vi "Init_graphe.vi"() -> ()   [LabVIEW 2013]
uses:
  <vilib>/Utility/miscctls.llb/LVRowAndColumnTypeDef.ctl
  <vilib>/Utility/file.llb/Read From Spreadsheet File (string).vi
panel:
  in  "Bouton Aide":bool
  in  "Quit":bool
  out "horodatage_ok":timestamp
  in  "Fichier données brutes":path
  out "Colonne données brutes":string="0"
  out "Ligne données brutes":string="0"
  out "Noms variables":string[](array[string])
  out "Séparateur fichier brute":string
  in  "Valider":bool
  in  "Nouveau format date":bool
  in  "Formats Date - Heure":string(combo)="\"%Y-%m-%d %H:%M:%S\""
  in  "Convertir Date  - heure":bool
  out "Nb lignes":i32
  in  "Séparateur":u16(ring)=1 items=["", ",", ";", ".", "Tab", "Espace"]
  out "Horodatage_1":timestamp[](array[timestamp]) format="%<%X\n%x>T"
  in  "Horodatage 2":timestamp
  out "Table":string[][](table)
  out "Donnees":dbl[][](array[numeric])
  in  "Bouton vide 2":bool
  # "Facultatif : \nSélectionner la dernière cellule des noms de variables  en appuyant sur la touche CTRL"
  # "Sélectionner la 1ère cellule\ndes noms de variables"
  # "Sélectionner la 1ère cellule\nd'horodatage"
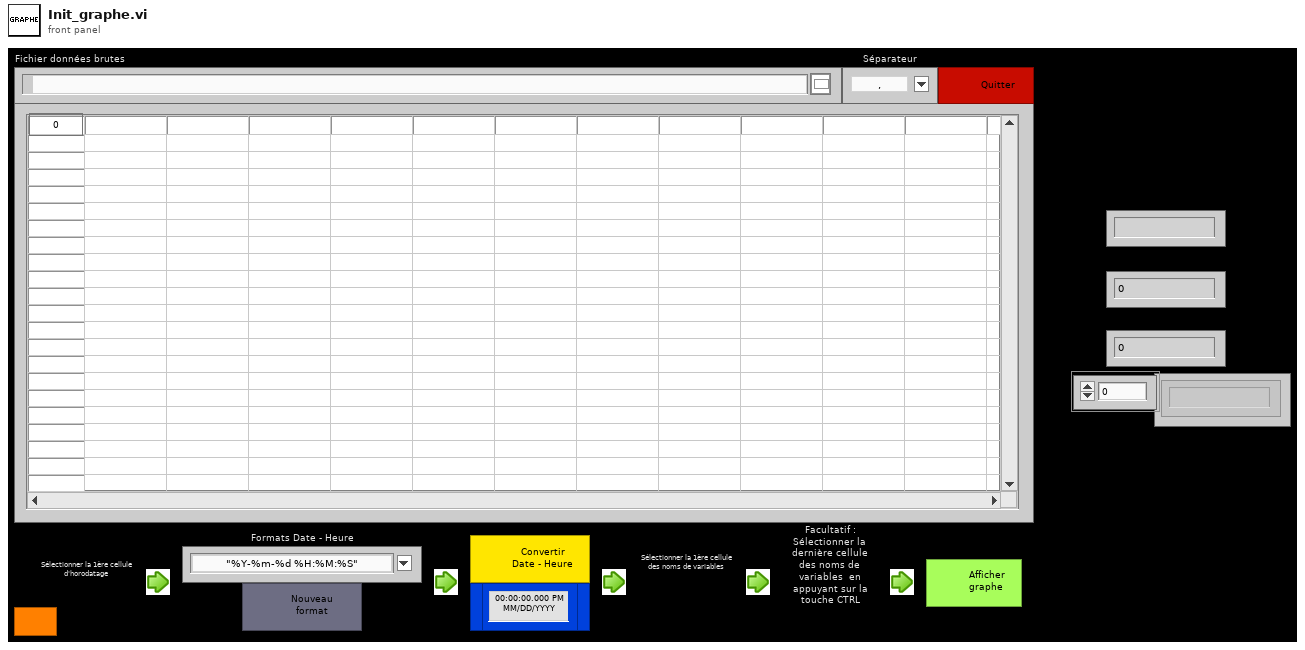
[diagram p1: front panel]
types:
  T1 = typedef "LVRowAndColumnTypeDef.ctl" = cluster{"Row":i32, "Column":i32}
  T2 = typedef "excel Object Reference.ctl" = refnum<k1>
  T3 = enum16{"Left Button", "Center Button", "Right Button", "Window Close"}
  T4 = cluster{"Shift":bool, "Ctrl":bool, "Alt":bool, "Cmd":bool, "Opt":bool}
  T5 = cluster{"Horodatage":timestamp[], "Donnees":dbl[]}[]
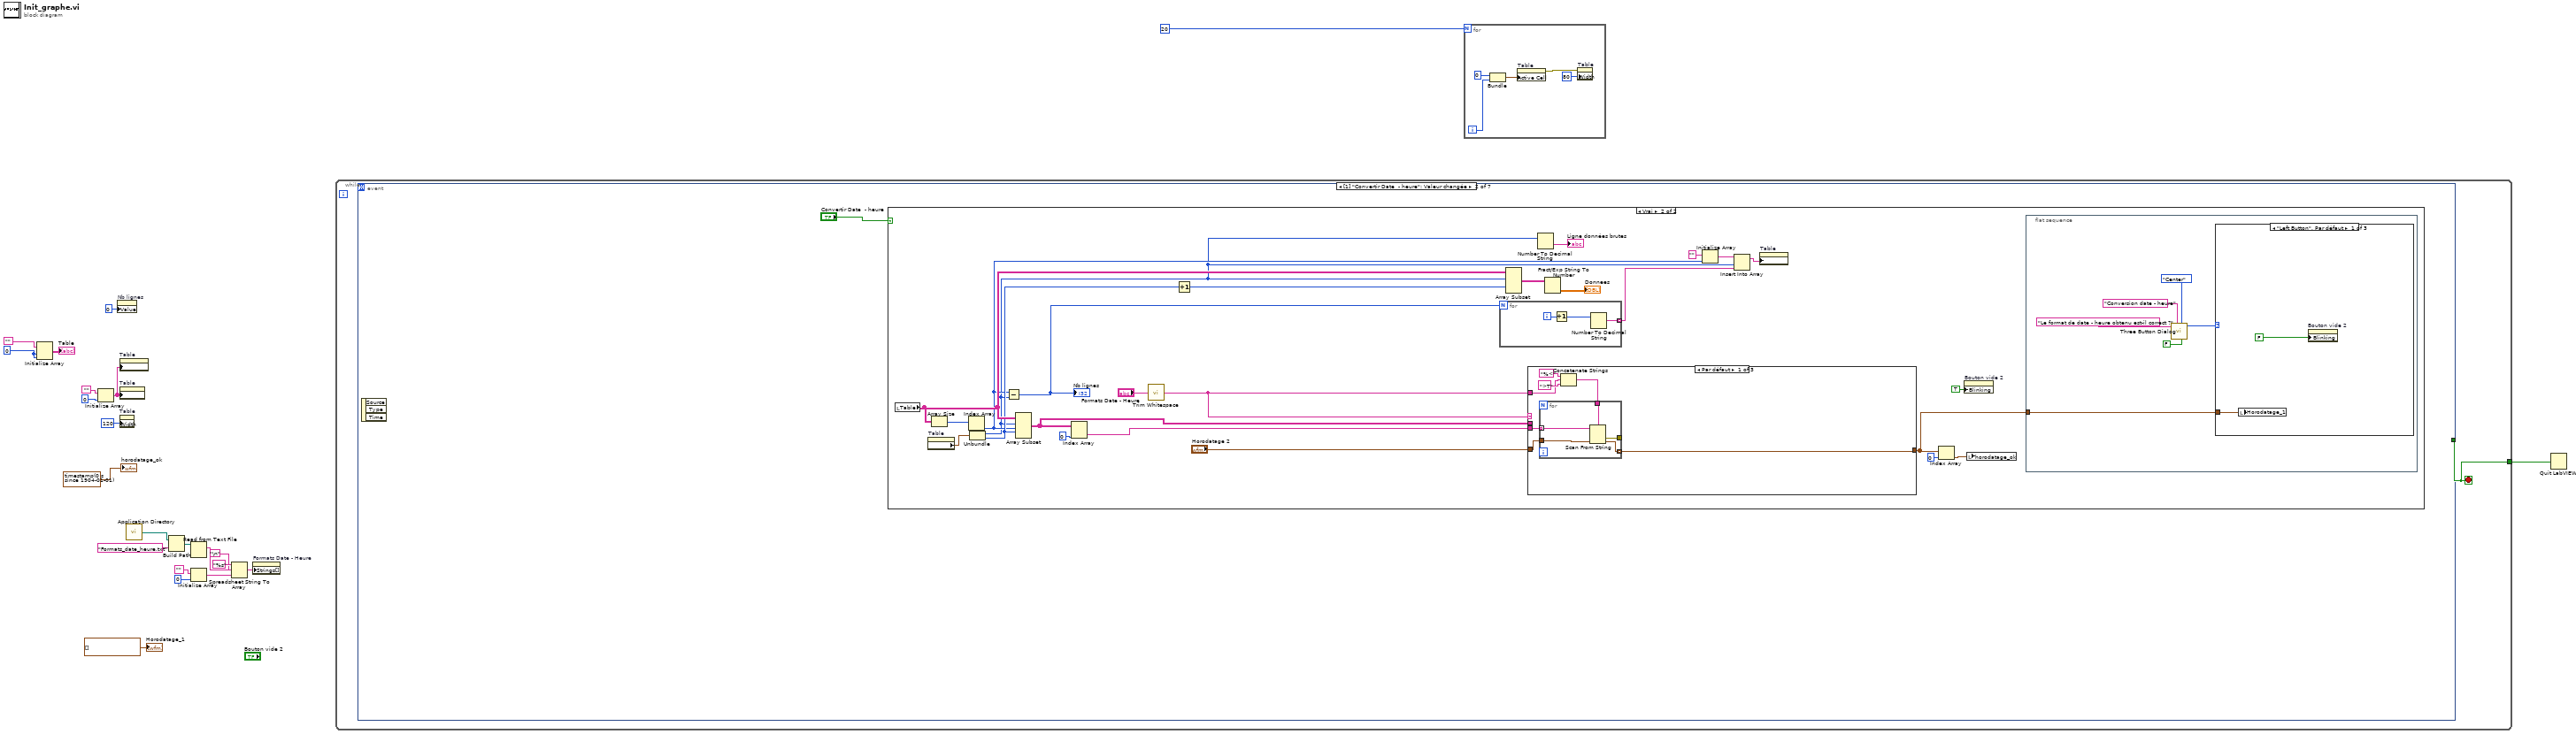
[diagram p0: block diagram]
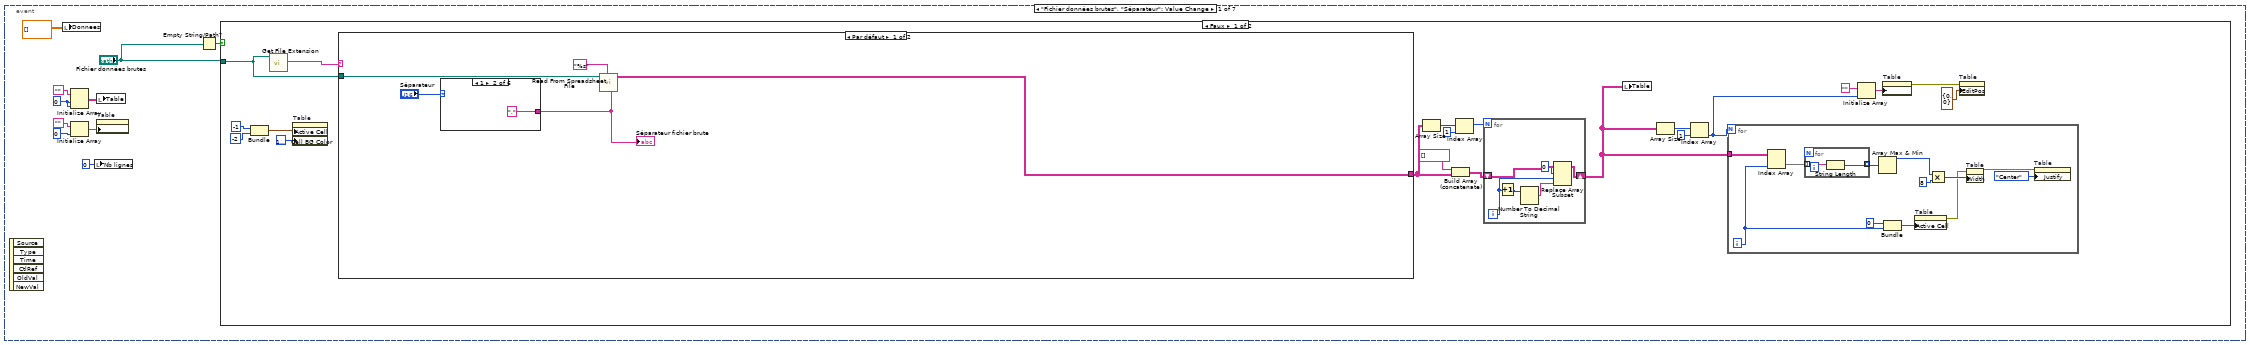
[diagram p2: hidden frame]
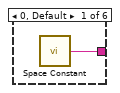
[diagram p3: hidden frame]
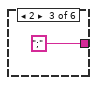
[diagram p4: hidden frame]
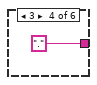
[diagram p5: hidden frame]
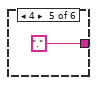
[diagram p6: hidden frame]
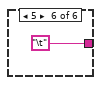
[diagram p7: hidden frame]
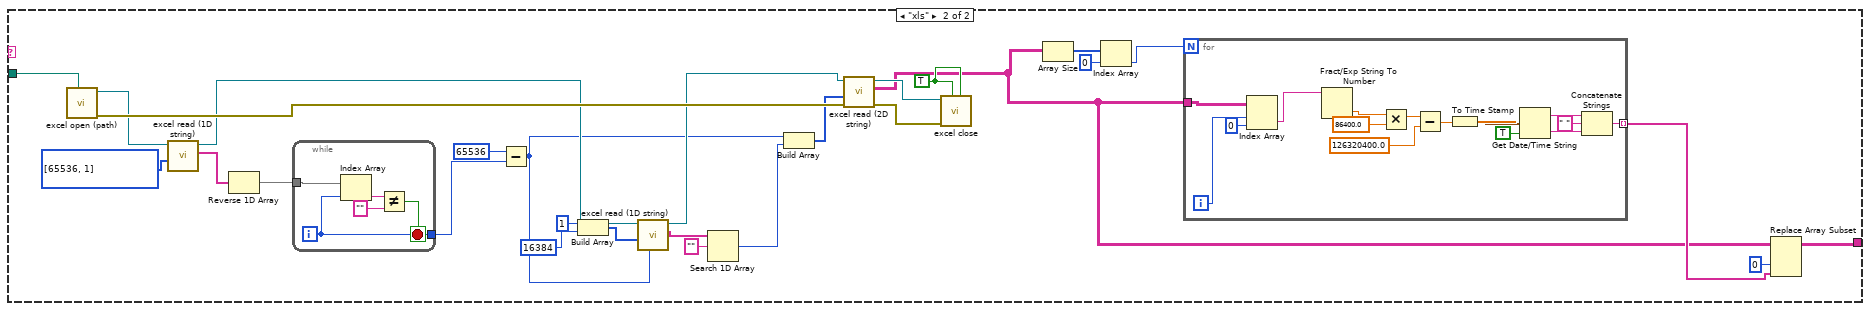
[diagram p8: hidden frame]
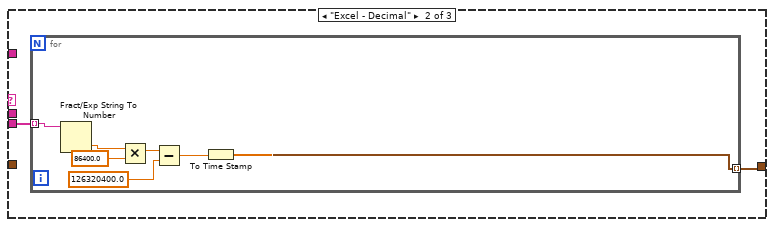
[diagram p13: hidden frame]
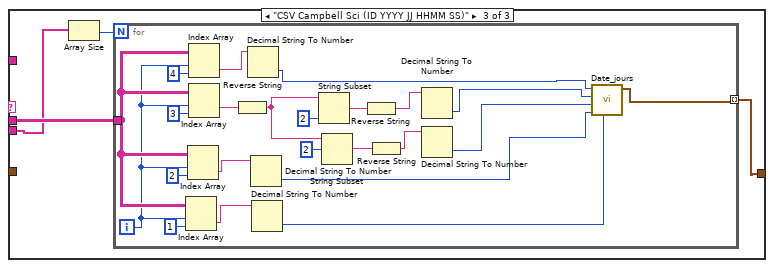
[diagram p14: hidden frame]
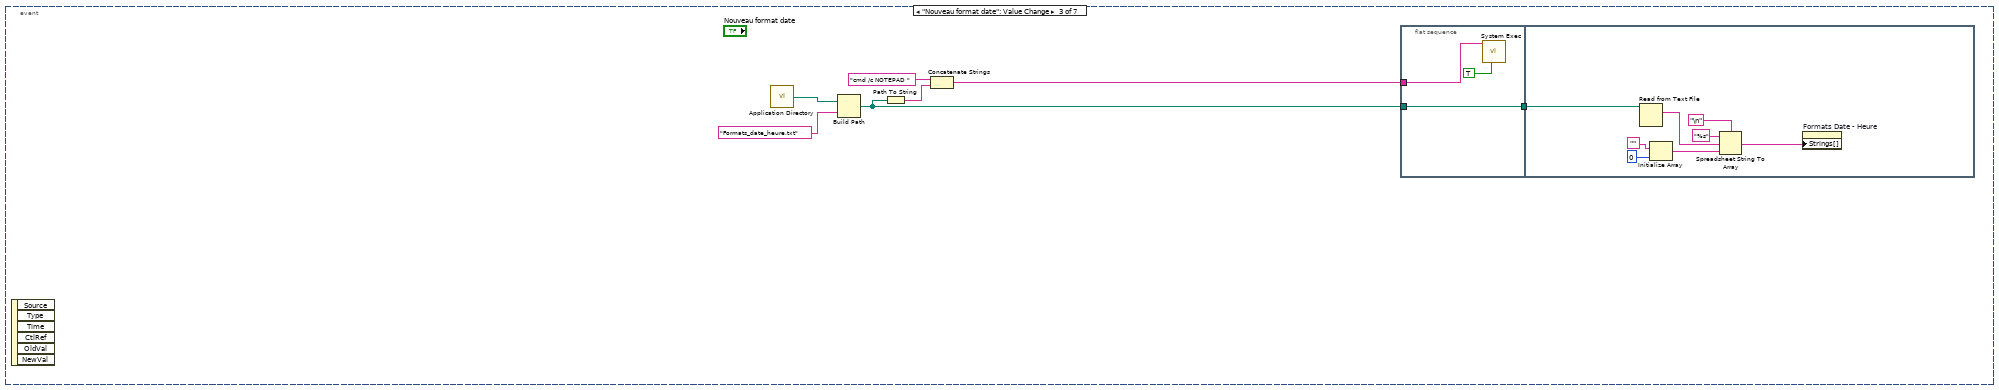
[diagram p15: hidden frame]
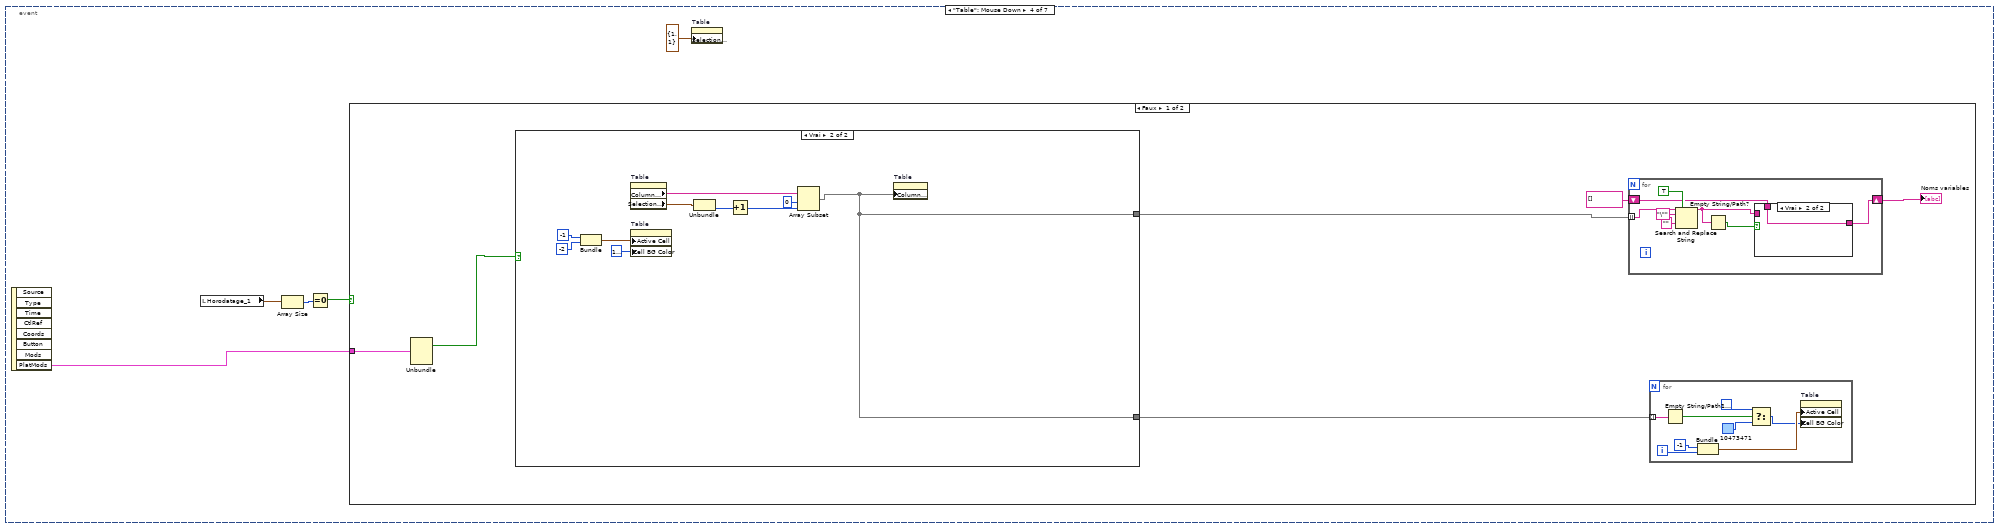
[diagram p16: hidden frame]
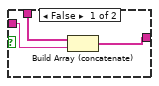
[diagram p17: hidden frame]
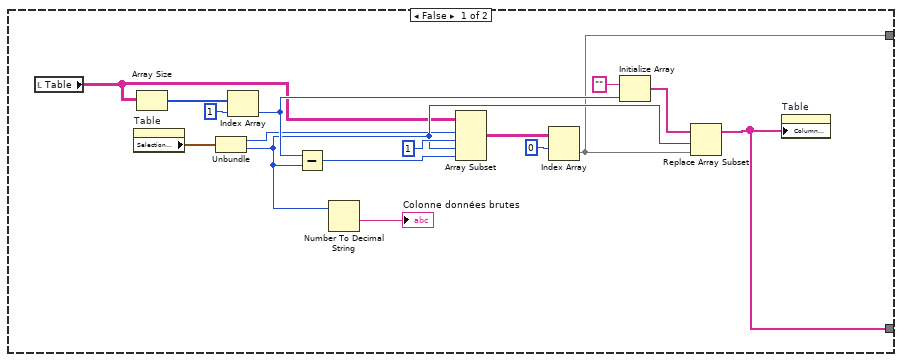
[diagram p18: hidden frame]
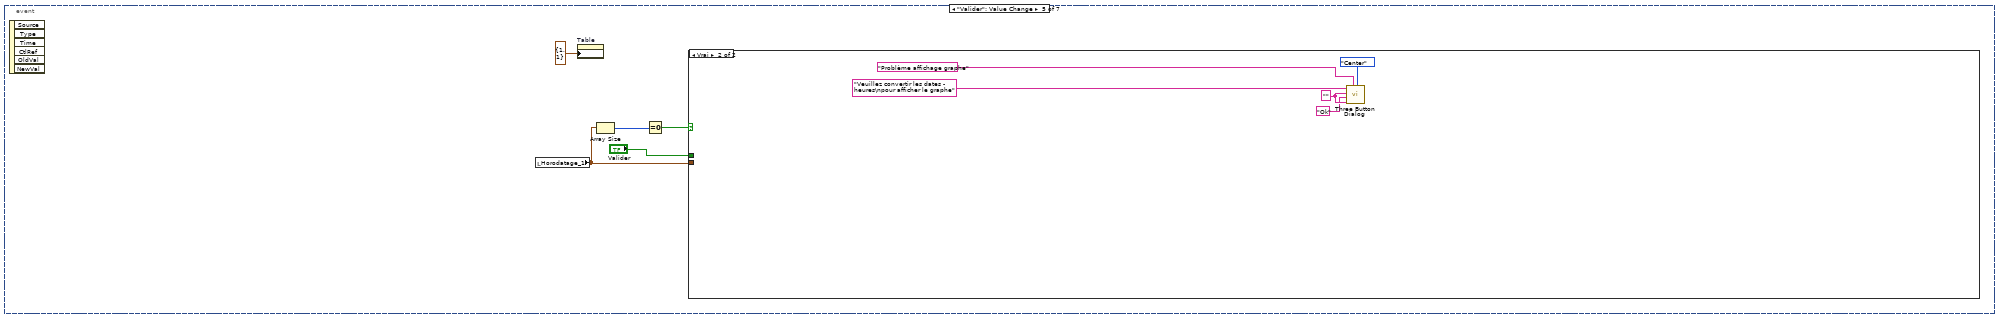
[diagram p20: hidden frame]
diagram:
  w4 = 0 ("taille de la dimension")
  n1 = Initialize Array("", w4, w4) -> (→"Table":string[][])
  n2 = Initialize Array("", 0 ("taille de la dimension")) -> (w11:string[])
  n3 = property on="Nb lignes" class="NumNb (strict)"("Value"=0 ("Nb lignes")) -> ()  [unwired: 2 in, 2 out]
  n4 = property on="Table" class="Tbl (strict)"("Row Headers[]"=w11) -> ()  [unwired: 2 in, 2 out]
  n5 = property on="Table" class="Tbl (strict)"("Column Headers[]"=w11) -> ()  [unwired: 2 in, 2 out]
  n6 = property on="Table" class="Tbl (strict)"("Width"=u32 120 ("Cellule active:Taille de la cellule:Largeur")) -> ()  [unwired: 2 in, 2 out]
  n7 = call <vilib>:"Application Directory.vi"() -> ("Application Directory"=w7:path)
  n8 = Build Path(base path=w7, name or relative path="Formats_date_heure.txt" ("nom ou chemin relatif")) -> (appended path=w15:path)
  n9 = Read from Text File(file (use dialog)=w15) -> (text=w20:string)  [unwired: 3 in, 3 out]
  n10 = Initialize Array("", 0 ("taille de la dimension")) -> (w16:string[])
  n11 = Spreadsheet String To Array(delimiter (Tab)="\n", format string="%s" ("chaîne de format"), spreadsheet string=w20, array type (2D Dbl)=w16) -> (array=w12:string[])
  n12 = property on="Formats Date - Heure" class="ChneDér"("Strings[]"=w12) -> ()  [unwired: 2 in, 2 out]
  n13 = while {
    tunnel: [w23] -> w1
    stop <- w23 stop-if-true
    n14 = event shown="[1] \"Convertir Date  - heure\": Valeur changée" {
      selector: _ -> [_ _ _ _ _ _ _]
      dyn-events: _ -> [_ _ _ _ _ _ _]
      timeout: _ -> [_ _ _ _ _ _ _]
      tunnel: [_ _ _ _ _ w324 _] -> w23
      event "Fichier données brutes", "Séparateur": Value Change {
        w33 = 0 ("taille de la dimension")
        n15 = event-data() -> ()  [unwired: 1 in, 6 out]
        n16 = local write "Donnees"(dbl[][] [] ("Donnees")) -> ()
        n17 = Initialize Array("", w33, w33) -> (w31:string[][])
        n18 = Initialize Array("", 0 ("taille de la dimension")) -> (w28:string[])
        n19 = local write "Nb lignes"(0 ("Nb lignes")) -> ()
        n20 = local write "Table"(w31) -> ()
        n21 = property on="Table" class="Tbl (strict)"("Row Headers[]"=w28) -> ()  [unwired: 2 in, 2 out]
        n22 = Empty String/Path?(string/path="Fichier données brutes") -> (empty?=w25:bool)
        n23 = case shown="Faux" w25 {
          tunnel: "Fichier données brutes" -> [w49 _]
          frame False {
            n24 = Bundle(-1, -2) -> (w44:cluster{i32, i32})  [unwired: 1 in]
            n25 = call <vilib>:"Get File Extension.vi"("file"=w49) -> ("lowercase file extension"=w48:string)  [unwired: 7 in, 3 out]
            n26 = property on="Table" class="Tbl (strict)"("Active Cell"=w44, "Cell BG Color"=u32 16777225) -> ()  [unwired: 2 in, 2 out]
            n27 = case shown="Par défaut" w48 {
              tunnel: w49 -> [w76 w112]
              tunnel: [w75 w85] -> w37
              frame Default {
                n28 = case shown="1" "Séparateur" {
                  tunnel: [w79 "," ";" "." "." "\t"] -> w74
                  frame 0, Default {
                    n29 = call <vilib>:"Space Constant.vi"() -> ("String"=w79:string)
                  }
                  frame 1 {
                  }
                  frame 2 {
                  }
                  frame 3 {
                  }
                  frame 4 {
                  }
                  frame 5 {
                  }
                }
                "Séparateur fichier brute" <- w74
                n30 = call-poly <vilib>:"Read From Spreadsheet File.vi"("delimiter (\\t)"=w74, "format (%s)"="%s", "file path (dialog if empty)"=w76) -> ("all rows"=w75:string[][])  [unwired: 4 in, 4 out]
              }
              frame "xls" {
                w108 = TRUE ("Override closing behavior")
                n31 = call <userlib>:"excel open (path).vi"("workbook path"=w112) -> ("error out"=w109:errorcluster, "reference"=w107:T2)  [unwired: 9 in]
                n32 = call <userlib>:"excel read (1D string).vi"("array size\n  - #rows\n  - #columns"=i32[] [65536, 1] ("array size\n  - #rows\n  - #columns"), "reference"=w107) -> ("1D String Array"=w105:string[], "duplicate reference"=w98:T2)  [unwired: 7 in, 1 out]
                n33 = Reverse 1D Array(array=w105) -> (reversed array=w103:string[])
                n34 = while {
                  tunnel: w103 -> [w132]
                  tunnel: [w128] -> w102
                  i -> [w128]
                  stop <- w129 stop-if-true
                  n35 = Index Array(array=w132, index=w128) -> (element=w131:string)
                  n36 = Not Equal?(x=w131, y="") -> (x != y?=w129:bool)
                }
                n37 = Subtract(x=65536, y=w102) -> (x-y=w95:i32)
                n38 = Build Array(1 ("élément"), 16384 ("élément")) -> (w99:i32[])
                n39 = call <userlib>:"excel read (1D string).vi"("Row"=w95, "array size\n  - #rows\n  - #columns"=w99, "reference"=w98) -> ("1D String Array"=w94:string[], "duplicate reference"=w97:T2)  [unwired: 6 in, 1 out]
                n40 = Search 1D Array(1D array=w94, element="" ("élément")) -> (index of element=w92:i32)  [unwired: 1 in]
                n41 = Build Array(w95, w92) -> (w104:i32[])
                n42 = call <userlib>:"excel read (2D string).vi"("error in (no error)"=w109, "array size\n  - #rows\n  - #columns"=w104, "reference"=w97) -> ("error out"=w110:errorcluster, "2D String Array"=w86:string[][], "duplicate reference"=w111:T2)  [unwired: 6 in]
                n43 = call <userlib>:"excel close.vi"("Close"=w108, "Override closing behavior"=w108, "error in (no error)"=w110, "reference"=w111) -> ()  [unwired: 7 in, 1 out]
                n44 = Array Size(array=w86) -> (size(s)=w88:i32[])
                n45 = Index Array(array=w88, index=0 ("indice")) -> (element=w89:i32)
                n46 = for {
                  N: w89 -> [_]
                  tunnel: w86 -> [w127]
                  tunnel: [w113] -> w91 mode=indexing
                  i -> [w126]
                  n47 = Index Array(array=w127, index (row)=w126, index (col)=0 ("indice désactivé (col)")) -> (element=w114:string)
                  n48 = Fract/Exp String To Number(string=w114) -> (number=w124:dbl)  [unwired: 3 in, 1 out]
                  n49 = Multiply(x=w124, y=86400.0) -> (x*y=w122:dbl)
                  n50 = Subtract(x=w122, y=126320400.0) -> (x-y=w120:dbl)
                  n51 = To Time Stamp(1:w120) -> (0:w119:timestamp)
                  n52 = Get Date/Time String(seconds (now)=w119, want seconds? (F)=TRUE ("secondes ? (F)")) -> (date string=w117:string, time string=w115:string)  [unwired: 1 in]
                  n53 = Concatenate Strings(w117, " " ("chaîne"), w115) -> (w113:string)
                }
                n54 = Replace Array Subset(array=w86, new element=w91, index (col)=0 ("indice désactivé (col)")) -> (w85:string[][])  [unwired: 1 in]
              }
            }
            n55 = Array Size(array=w37) -> (size(s)=w39:i32[])
            n56 = Build Array (concatenate)(string[] [] ("élément"), w37) -> (w35:string[][])
            n57 = Index Array(array=w39, index=1 ("indice")) -> (element=w38:i32)
            n58 = for {
              N: w38 -> [_]
              shift-right: [w59] -> w41
              shift-left: w35 -> [w58]
              i -> [w55]
              n59 = Increment(x=w55) -> (x+1=w57:i32)
              n60 = Number To Decimal String(number=w57) -> (decimal integer string=w54:string)  [unwired: 1 in]
              n61 = Replace Array Subset(array=w58, new element=w54, index (row)=0 ("indice désactivé (ligne)"), index (col)=w55) -> (w59:string[][])
            }
            n62 = local write "Table"(w41) -> ()
            n63 = Array Size(array=w41) -> (size(s)=w47:i32[])
            n64 = Index Array(array=w47, index=1 ("indice")) -> (element=w34:i32)
            n65 = for {
              N: w34 -> [_]
              tunnel: w41 -> [w71]
              i -> [w63]
              n66 = Index Array(array=w71, index (col)=w63) -> (element=w68:string[])  [unwired: 1 in]
              n67 = for {
                tunnel: w68 -> [w73] mode=indexing
                tunnel: [w72] -> w67 mode=indexing
                n68 = String Length(string=w73) -> (length=w72:i32)
              }
              n69 = Array Max & Min(array=w67) -> (max value=w66:i32)  [unwired: 3 out]
              n70 = Bundle(0, w63) -> (w65:cluster{i32, i32})  [unwired: 1 in]
              n71 = property on="Table" class="Tbl (strict)"("Active Cell"=w65) -> (error out=w64:errorcluster)  [unwired: 2 in, 1 out]
              n72 = Multiply(x=w66, y=8) -> (x*y=w70:i32)
              n73 = property on="Table" class="Tbl (strict)"(error in=w64, "Width"=w70) -> (error out=w61:errorcluster)  [unwired: 1 in, 1 out]
              n74 = property on="Table" class="Tbl (strict)"(error in=w61, "Justify"=enum16{"Left", "Center", "Right"}."Center" ("Cellule active:Justification de la cellule")) -> ()  [unwired: 1 in, 2 out]
            }
            n75 = Initialize Array("", w34) -> (w52:string[])
            n76 = property on="Table" class="Tbl (strict)"("Column Headers[]"=w52) -> (error out=w50:errorcluster)  [unwired: 2 in, 1 out]
            n77 = property on="Table" class="Tbl (strict)"(error in=w50, "EditPos"=T1 {"Row"=0, "Column"=0} ("Cellule active:Cellule active")) -> ()  [unwired: 1 in, 2 out]
          }
          frame True {
          }
        }
      }
      event "Convertir Date  - heure": Value Change {
        n78 = event-data() -> ()  [unwired: 1 in, 3 out]
        n79 = case shown="Vrai" "Convertir Date  - heure" {
          frame False {
          }
          frame True {
            n80 = local read "Table"() -> (w153:string[][])
            n81 = property on="Table" class="Tbl (strict)"() -> ("Selection Start"=w156:T1)  [unwired: 2 in, 2 out]
            n82 = Array Size(array=w153) -> (size(s)=w154:i32[])
            n83 = Index Array(array=w154) -> (element=w147:i32)  [unwired: 1 in]
            n84 = Unbundle(w156) -> ("Row"=w143:i32, "Column"=w148:i32)
            n85 = Subtract(x=w147, y=w143) -> (x-y=w138:i32)
            "Nb lignes" <- w138
            n86 = Array Subset(array=w153, index (row)=w143, length (row)=w147, index (col)=w148) -> (w140:string[][])  [unwired: 1 in]
            n87 = Index Array(array=w140, index (col)=0 ("indice (ligne)")) -> (element=w145:string[])  [unwired: 1 in]
            n88 = call <vilib>:"Trim Whitespace.vi"("string"="Formats Date - Heure") -> ("trimmed string"=w134:string)  [unwired: 1 in]
            n89 = Increment(x=w148) -> (x+1=w155:i32)
            n90 = for {
              N: w138 -> [_]
              tunnel: [w216] -> w150 mode=indexing
              i -> [w217]
              n91 = Increment(x=w217) -> (x+1=w215:i32)
              n92 = Number To Decimal String(number=w215) -> (decimal integer string=w216:string)  [unwired: 1 in]
            }
            n93 = Array Subset(array=w153, index (row)=w143, index (col)=w155) -> (w157:string[][])  [unwired: 2 in]
            n94 = case shown="Par défaut" w134 {
              tunnel: "Horodatage 2" -> [w173 _ _]
              tunnel: w145 -> [w170 w180 w188]
              tunnel: [w169 w179 w190] -> w137
              tunnel: w134 -> [w167 _ _]
              tunnel: w140 -> [_ _ w191]
              frame Default {
                n95 = Concatenate Strings("%<", w167, ">T") -> (w168:string)
                n96 = for {
                  tunnel: [w178] -> w169 mode=indexing
                  tunnel: w173 -> [w177]
                  tunnel: w168 -> [w176]
                  tunnel: w170 -> [w174] mode=indexing
                  tunnel: [w175] -> _
                  n97 = Scan From String(format string=w176, input string=w174, default 1=w177) -> (error out=w175:errorcluster, output 1=w178:timestamp)  [unwired: 2 in, 2 out]
                }
              }
              frame "Excel - Decimal" {
                n98 = for {
                  tunnel: [w181] -> w179 mode=indexing
                  tunnel: w180 -> [w187] mode=indexing
                  n99 = Fract/Exp String To Number(string=w187) -> (number=w186:dbl)  [unwired: 3 in, 1 out]
                  n100 = Multiply(x=w186, y=86400.0) -> (x*y=w184:dbl)
                  n101 = Subtract(x=w184, y=126320400.0) -> (x-y=w182:dbl)
                  n102 = To Time Stamp(1:w182) -> (0:w181:timestamp)
                }
              }
              frame "CSV Campbell Sci (ID YYYY JJ HHMM SS)" {
                n103 = Array Size(array=w188) -> (size(s)=w189:i32)
                n104 = for {
                  N: w189 -> [_]
                  tunnel: w191 -> [w201]
                  tunnel: [w192] -> w190 mode=indexing
                  i -> [w200]
                  n105 = Index Array(array=w201, index (row)=w200, index (col)=1 ("indice désactivé (col)")) -> (element=w198:string)
                  n106 = Index Array(array=w201, index (row)=w200, index (col)=2 ("indice désactivé (col)")) -> (element=w199:string)
                  n107 = Index Array(array=w201, index (row)=w200, index (col)=4 ("indice désactivé (col)")) -> (element=w213:string)
                  n108 = Index Array(array=w201, index (row)=w200, index (col)=3 ("indice désactivé (col)")) -> (element=w211:string)
                  n109 = Reverse String(1:w211) -> (0:w207:string)
                  n110 = Decimal String To Number(string=w213) -> (number=w197:i32)  [unwired: 2 in, 1 out]
                  n111 = Decimal String To Number(string=w199) -> (number=w194:i32)  [unwired: 2 in, 1 out]
                  n112 = Decimal String To Number(string=w198) -> (number=w193:i32)  [unwired: 2 in, 1 out]
                  n113 = String Subset(string=w207, length (rest)=2 ("longueur (reste)")) -> (substring=w209:string)  [unwired: 1 in]
                  n114 = String Subset(string=w207, offset (0)=2) -> (substring=w205:string)  [unwired: 1 in]
                  n115 = Reverse String(1:w209) -> (0:w208:string)
                  n116 = Reverse String(1:w205) -> (0:w204:string)
                  n117 = Decimal String To Number(string=w208) -> (number=w196:i32)  [unwired: 2 in, 1 out]
                  n118 = Decimal String To Number(string=w204) -> (number=w195:i32)  [unwired: 2 in, 1 out]
                  n119 = call "Date_jours.vi"("year"=w193, "jours n"=w194, "hour"=w195, "minute"=w196, "second"=w197) -> ("horodatage"=w192:timestamp)  [unwired: 6 in]
                }
              }
            }
            n120 = Number To Decimal String(number=w143) -> (decimal integer string=→"Ligne données brutes":string)  [unwired: 1 in]
            n121 = Fract/Exp String To Number(string=w157) -> (number=→"Donnees":dbl[][])  [unwired: 3 in, 1 out]
            n122 = Initialize Array("", w147) -> (w151:string[])
            n123 = Insert Into Array(array=w151, index=w143, new element=w150) -> (w139:string[])
            n124 = property on="Table" class="Tbl (strict)"("Row Headers[]"=w139) -> ()  [unwired: 2 in, 2 out]
            n125 = Index Array(array=w137, index=0 ("indice")) -> (element=w136:timestamp)
            n126 = property on="Bouton vide 2" class="Bool"("Blinking"=TRUE ("Clignotant")) -> ()  [unwired: 2 in, 2 out]
            n127 = local write "horodatage_ok"(w136) -> ()
            n128 = flat-sequence {
              tunnel: w137 -> [w159]
              frame #0 {
                n129 = call <vilib>:"Three Button Dialog.vi"("Allow user to close window? (TRUE)"=FALSE, "Justify Message (Left)"=enum16{"Left", "Center", "Right"}."Center", "Window Title (\"\")"="Conversion date - heure" ("error source (\" \")"), "message"="Le format de date - heure obtenu est-il correct ?" ("error source (\" \")")) -> ("Which Button?"=w162:T3)  [unwired: 7 in]
                n130 = case shown="\"Left Button\", Par défaut" w162 {
                  tunnel: w159 -> [w166 _ _]
                  frame "Left Button", Default {
                    n131 = local write "Horodatage_1"(w166) -> ()
                    n132 = property on="Bouton vide 2" class="Bool"("Blinking"=FALSE ("Clignotant")) -> ()  [unwired: 2 in, 2 out]
                  }
                  frame "Center Button" {
                  }
                  frame "Right Button" {
                  }
                }
              }
            }
          }
        }
      }
      event "Nouveau format date": Value Change {
        n133 = event-data() -> ()  [unwired: 1 in, 6 out]
        n134 = call <vilib>:"Application Directory.vi"() -> ("Application Directory"=w218:path)
        n135 = Build Path(base path=w218, name or relative path="Formats_date_heure.txt" ("nom ou chemin relatif")) -> (appended path=w220:path)
        n136 = Path To String(path=w220) -> (string=w221:string)
        n137 = Concatenate Strings("cmd /c NOTEPAD " ("command line"), w221) -> (w223:string)
        n138 = flat-sequence {
          tunnel: w223 -> [w227]
          tunnel: w220 -> [w225]
          tunnel: [w225] -> w219
          tunnel: w219 -> [w228]
          frame #0 {
            n139 = call <vilib>:"System Exec.vi"("run minimized? (F)"=TRUE, "command line"=w227) -> ()  [unwired: 6 in, 4 out]
          }
          frame #1 {
            n140 = Read from Text File(file (use dialog)=w228) -> (text=w229:string)  [unwired: 3 in, 3 out]
            n141 = Initialize Array("", 0 ("taille de la dimension")) -> (w233:string[])
            n142 = Spreadsheet String To Array(delimiter (Tab)="\n", format string="%s" ("chaîne de format"), spreadsheet string=w229, array type (2D Dbl)=w233) -> (array=w235:string[])
            n143 = property on="Formats Date - Heure" class="ChneDér"("Strings[]"=w235) -> ()  [unwired: 2 in, 2 out]
          }
        }
      }
      event "Table": Mouse Down {
        n144 = event-data() -> ("PlatMods"=w239:T4)  [unwired: 1 in, 7 out]
        n145 = local read "Horodatage_1"() -> (w238:timestamp[])
        n146 = Array Size(array=w238) -> (size(s)=w237:i32)
        n147 = Equal To 0?(x=w237) -> (x = 0?=w236:bool)
        n148 = case shown="Faux" w236 {
          tunnel: w239 -> [w246 _]
          frame False {
            n149 = Unbundle(w246) -> ("Ctrl"=w245:bool)  [unwired: 4 out]
            n150 = case shown="Vrai" w245 {
              tunnel: [w270 w289] -> w242
              tunnel: [w268 w289] -> w241
              frame False {
                n151 = local read "Table"() -> (w267:string[][])
                n152 = property on="Table" class="Tbl (strict)"() -> ("Selection Start"=w269:T1)  [unwired: 2 in, 2 out]
                n153 = Array Size(array=w267) -> (size(s)=w280:i32[])
                n154 = Unbundle(w269) -> ("Row"=w271:i32, "Column"=w273:i32)
                n155 = Index Array(array=w280, index=1 ("indice")) -> (element=w274:i32)
                n156 = Subtract(x=w274, y=w273) -> (x-y=w278:i32)
                n157 = Number To Decimal String(number=w273) -> (decimal integer string=→"Colonne données brutes":string)  [unwired: 1 in]
                n158 = Array Subset(array=w267, index (row)=w271, length (row)=1 ("longueur"), index (col)=w273, length (col)=w278) -> (w281:string[][])
                n159 = Index Array(array=w281, index (row)=0 ("indice (ligne)")) -> (element=w270:string[])  [unwired: 1 in]
                n160 = Initialize Array("", w274) -> (w276:string[])
                n161 = Replace Array Subset(array=w276, new element=w270, index=w273) -> (w268:string[])
                n162 = property on="Table" class="Tbl (strict)"("Column Headers[]"=w268) -> ()  [unwired: 2 in, 2 out]
              }
              frame True {
                n163 = Bundle(-1, -2) -> (w286:cluster{i32, i32})  [unwired: 1 in]
                n164 = property on="Table" class="Tbl (strict)"() -> ("Column Headers[]"=w288:string[], "Selection Start"=w283:T1)  [unwired: 2 in, 2 out]
                n165 = property on="Table" class="Tbl (strict)"("Active Cell"=w286, "Cell BG Color"=u32 16777225) -> ()  [unwired: 2 in, 2 out]
                n166 = Unbundle(w283) -> ("Column"=w290:i32)  [unwired: 1 out]
                n167 = Increment(x=w290) -> (x+1=w292:i32)
                n168 = Array Subset(array=w288, index=0 ("indice"), length=w292) -> (w289:string[])
                n169 = property on="Table" class="Tbl (strict)"("Column Headers[]"=w289) -> ()  [unwired: 2 in, 2 out]
              }
            }
            n170 = for {
              tunnel: w242 -> [w255] mode=indexing
              shift-right: [w257] -> w244
              shift-left: string[] [] -> [w258]
              n171 = Search and Replace String(replace all?=TRUE ("tout remplacer ? (F)"), input string=w255, search string="\"" ("chaîne recherchée"), replace string="" ("chaîne de remplacement (\"\")")) -> (result string=w256:string)  [unwired: 4 in, 3 out]
              n172 = Empty String/Path?(string/path=w256) -> (empty?=w259:bool)
              n173 = case shown="Vrai" w259 {
                tunnel: w258 -> [w265 w266]
                tunnel: [w263 w266] -> w257
                tunnel: w256 -> [w264 _]
                frame False {
                  n174 = Build Array (concatenate)(w265, w264) -> (w263:string[])
                }
                frame True {
                }
              }
            }
            "Noms variables" <- w244
            n175 = for {
              tunnel: w241 -> [w254] mode=indexing
              i -> [w252]
              n176 = Empty String/Path?(string/path=w254) -> (empty?=w250:bool)
              n177 = Bundle(-1, w252) -> (w251:cluster{i32, i32})  [unwired: 1 in]
              n178 = Select(t=u32 16777225, s=w250, f=u32 10473471) -> (s? t:f=w247:u32)
              n179 = property on="Table" class="Tbl (strict)"("Active Cell"=w251, "Cell BG Color"=w247) -> ()  [unwired: 2 in, 2 out]
            }
          }
          frame True {
          }
        }
        n180 = property on="Table" class="Tbl (strict)"("Selection Size"=T1 {"Row"=1, "Column"=1} ("Taille de sélection")) -> ()  [unwired: 2 in, 2 out]
      }
      event "Valider": Value Change {
        n181 = event-data() -> ()  [unwired: 1 in, 6 out]
        n182 = local read "Horodatage_1"() -> (w296:timestamp[])
        n183 = property on="Table" class="Tbl (strict)"("Selection Size"=T1 {"Row"=1, "Column"=1} ("Taille de sélection")) -> ()  [unwired: 2 in, 2 out]
        n184 = Array Size(array=w296) -> (size(s)=w295:i32)
        n185 = Equal To 0?(x=w295) -> (x = 0?=w294:bool)
        n186 = case shown="Vrai" w294 {
          tunnel: "Valider" -> [w299 _]
          tunnel: w296 -> [w298 _]
          frame False {
            n187 = case shown="Vrai" w299 {
              tunnel: w298 -> [_ w305]
              frame False {
              }
              frame True {
                n188 = local read "Table"() -> (w315:string[][])
                n189 = property on="Table" class="Tbl (strict)"() -> ("Selection Start"=w301:T1)  [unwired: 2 in, 2 out]
                n190 = Array Size(array=w315) -> (size(s)=w314:i32[])
                n191 = Unbundle(w301) -> ("Row"=w310:i32, "Column"=w309:i32)
                n192 = Index Array(array=w314, index=1 ("indice")) -> (element=w306:i32)
                n193 = Subtract(x=w306, y=w309) -> (x-y=w312:i32)
                n194 = Array Subset(array=w315, index (row)=w310, length (row)=1 ("longueur"), index (col)=w309, length (col)=w312) -> (w317:string[][])
                n195 = Index Array(array=w317, index (row)=0 ("indice (ligne)")) -> (element=w304:string[])  [unwired: 1 in]
                n196 = Initialize Array("", w306) -> (w308:string[])
                n197 = Replace Array Subset(array=w308, new element=w304, index=w309) -> ()  [unwired: 1 out]
                n198 = local read "Donnees"() -> (w316:dbl[][])
                n199 = property on="Table" class="Tbl (strict)"() -> ("Column Headers[]"=w300:string[])  [unwired: 2 in, 2 out]
                n200 = call "MAJ_Graphe.vi"("Horodatage"=w305, "Donnees"=w316, "Entetes colonnes"=w300) -> ("Graphe"=w303:T5, "Paramètres à afficher"=w302:string[])  [unwired: 5 in]
                n201 = call "Graphe_XY.vi"("Graphe"=w303, "Tableau de chaînes"=w302) -> ()  [unwired: 9 in]
              }
            }
          }
          frame True {
            w321 = "" ("Left Button Text (\"Yes\")")
            n202 = call <vilib>:"Three Button Dialog.vi"("Justify Message (Left)"=enum16{"Left", "Center", "Right"}."Center", "Window Title (\"\")"="Problème affichage graphe" ("Window Title (\"\")"), "Right Button Text (\"Cancel\")"=w321, "Center Button Text (\"No\")"="Ok" ("Center Button Text (\"No\")"), "Left Button Text (\"Yes\")"=w321, "message"="Veuillez convertir les dates - heures\npour afficher le graphe") -> ()  [unwired: 5 in, 1 out]
          }
        }
      }
      event "Quit": Value Change {
        n203 = event-data() -> ("NewVal"=w324:bool)  [unwired: 1 in, 5 out]
      }
      event "Bouton Aide": Value Change {
        n204 = event-data() -> ()  [unwired: 1 in, 6 out]
        n205 = call <vilib>:"Application Directory.vi"() -> ("Application Directory"=w326:path)
        n206 = Build Path(base path=w326, name or relative path="Logiciel GRAPHE_Instruction.pdf" ("standard input")) -> (appended path=w325:path)
        n207 = call "Open PDF.vi"("Path"=w325) -> ()  [unwired: 5 in, 2 out]
      }
    }
  }
  n208 = for {
    N: 20 -> [_]
    i -> [w330]
    n209 = Bundle(0, w330) -> (w331:cluster{i32, i32})  [unwired: 1 in]
    n210 = property on="Table" class="Tbl (strict)"("Active Cell"=w331) -> (error out=w328:errorcluster)  [unwired: 2 in, 1 out]
    n211 = property on="Table" class="Tbl (strict)"(error in=w328, "Width"=u32 80 ("Cellule active:Taille de la cellule:Largeur")) -> ()  [unwired: 1 in, 2 out]
  }
  n212 = Quit LabVIEW(quit? (T)=w1) -> ()
  "Horodatage_1" <- timestamp[] [] ("Horodatage")
  "horodatage_ok" <- timestamp(0 s since 1904-01-01)
